vi "Actor Core_mouse down.vi"(8 "error in":errorcluster, 11 "Batch proc":refnum<class "Batch Processor.lvclass">) -> (0 "error out":errorcluster, 3 "Actor out":refnum<class "Actor.lvclass">)   [LabVIEW 2020]
doc: "LabActor main control pannel"
uses:
  <vilib>/ActorFramework/Actor/Actor.lvclass
  <vilib>/ActorFramework/Stop Msg/Stop Msg.lvclass
  LabActor Messages/Stop Measurements Command Msg/Stop Measurements Command Msg.lvclass
  Application Controller Messages/Open Waveform File Plot Msg/Open Waveform File Plot Msg.lvclass
  Plots/Plot types.ctl
  Template Module Messages/Save Configuration Msg/Save Configuration Msg.lvclass
  Template Module Messages/Restore Configuration Msg/Restore Configuration Msg.lvclass
  Batch Processor Messages/List Folder Files Msg/List Folder Files Msg.lvclass
  Batch Processor Messages/Start Batch Process Msg/Start Batch Process Msg.lvclass
  NHMFL_Core/Libraries/Queued Listbox/Queued Listbox.xctl
  Batch Processor Messages/Select Item Msg/Select Item Msg.lvclass
  Batch Processor.lvclass
  C:/GitHub/LabActor/Controllers/Application Controller/Application Controller.lvclass
  C:/GitHub/LabActor/Controllers/Process Controller/Process Controller.lvclass
  C:/GitHub/LabActor/Worker/Worker.lvclass
  C:/GitHub/LabActor/Template Module/Template Module.lvclass
  C:/Program Files/National Instruments/LabVIEW 2020/vi.lib/ActorFramework/Actor/Actor.lvclass
  C:/GitHub/LabActor/Controllers/Batch Processor/Batch Processor.lvclass
panel:
  in  "Add files  from m-file":bool
  in  "Clear files":bool
  in  "Add files":bool
  in  "Step Forward Button":bool
  out "Current file":u32
  out "Elapsed time":dbl format="%#_gs"
  in  "Configuration":T1
  in  "All files in folder":bool
  in  "About Button":bool
  in  "Clear log":bool
  out "Error log":string
  out "Monitor file":path caption="Monitor\nFile"
  in  "Exit":bool
  in  "Write cfg":bool
  in  "Read cfg":bool
  in  "View XY Plot":bool
  out "Monitor Running":bool
  in  "Stop monitor":bool
  in  "Start monitor":bool
  in  "Monitor":string[](xcontrol) caption="Processors"
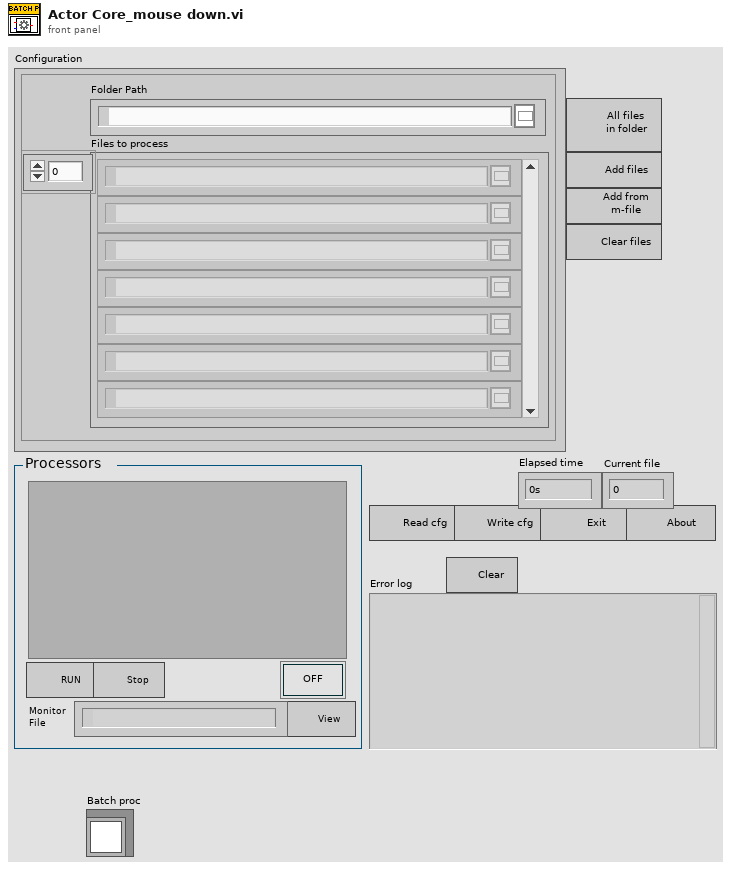
[diagram p1: front panel]
types:
  T1 = cluster{"Folder Path":path, "Files to process":path[]}
  T2 = typedef "Plot types.ctl" = enum16{"Waveform Plot", "XY Plot", "Full XY"}
  T3 = typedef "LVRectTypeDef.ctl" = cluster{"Left":i16, "Top":i16, "Right":i16, "Bottom":i16}
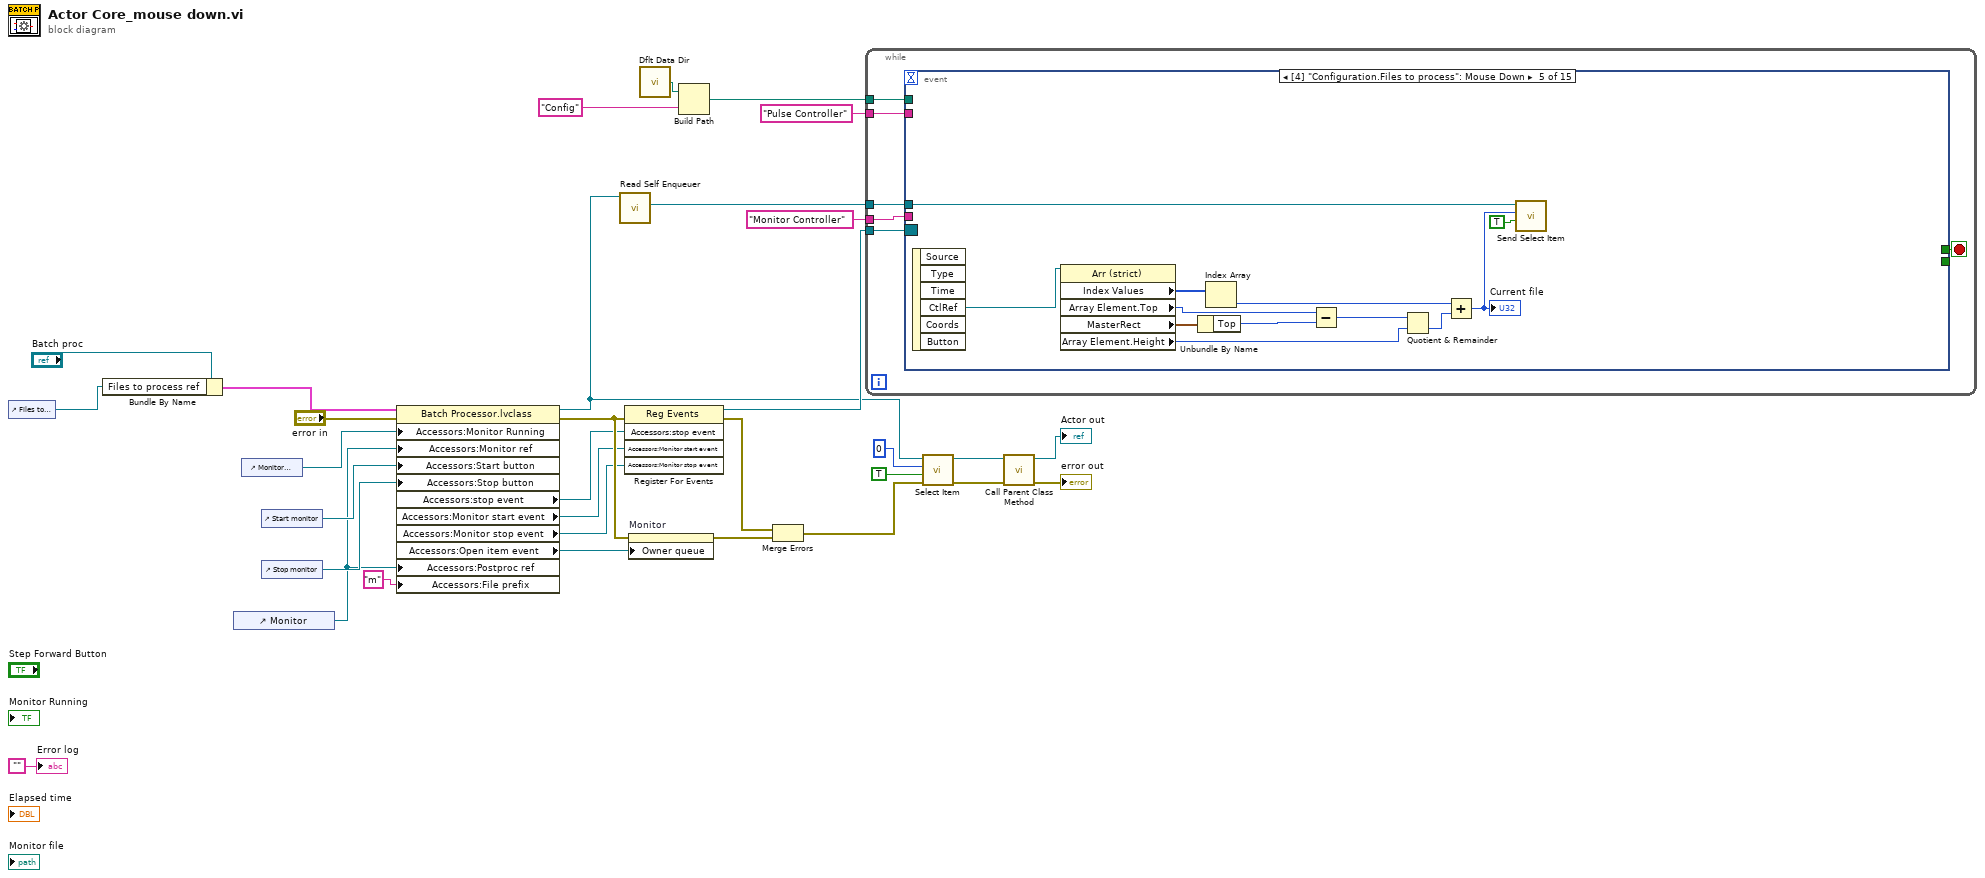
[diagram p0: block diagram]
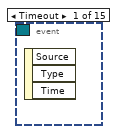
[diagram p2: hidden frame]
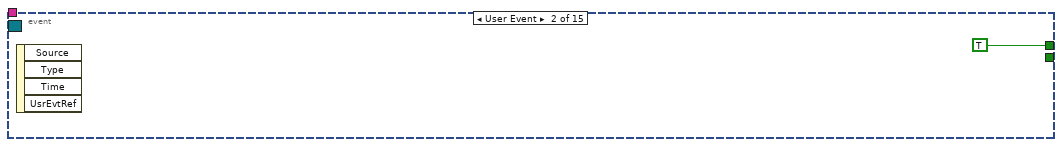
[diagram p3: hidden frame]
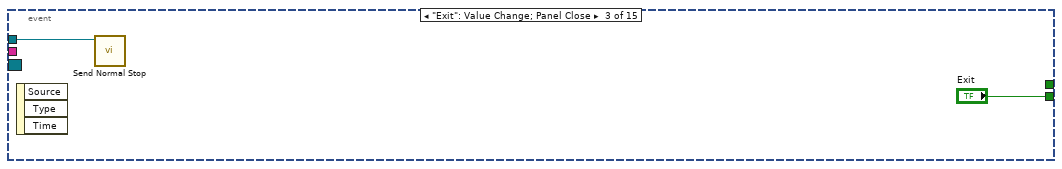
[diagram p4: hidden frame]
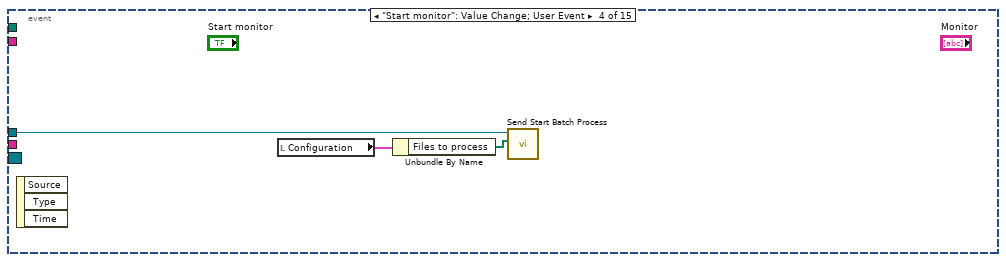
[diagram p5: hidden frame]
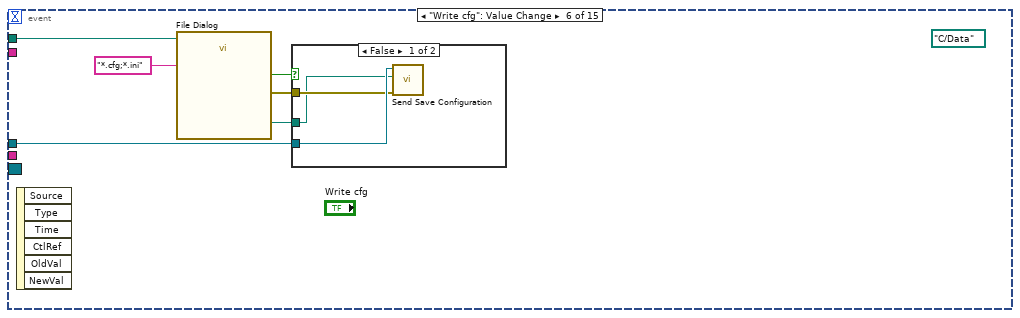
[diagram p6: hidden frame]
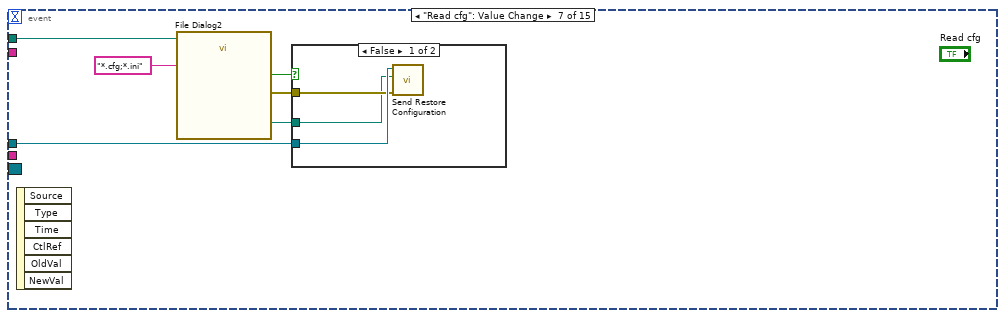
[diagram p8: hidden frame]
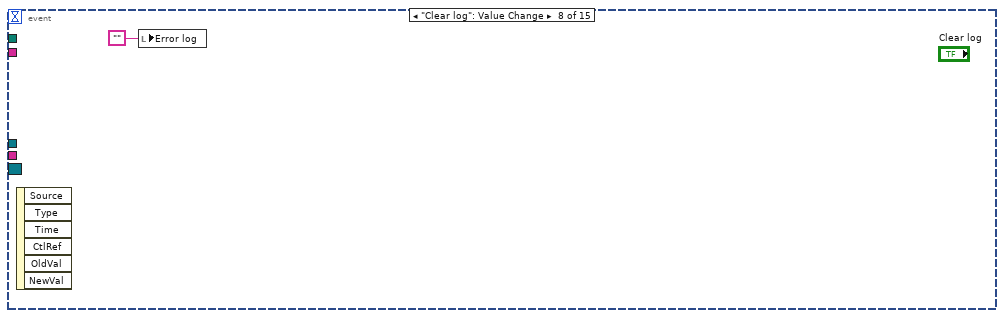
[diagram p10: hidden frame]
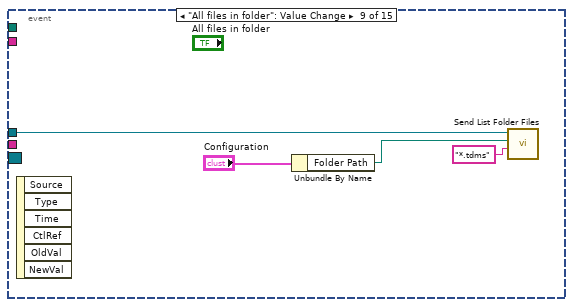
[diagram p11: hidden frame]
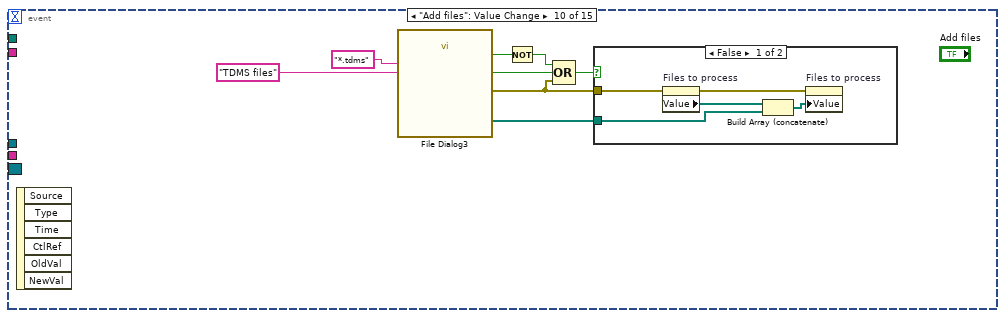
[diagram p12: hidden frame]
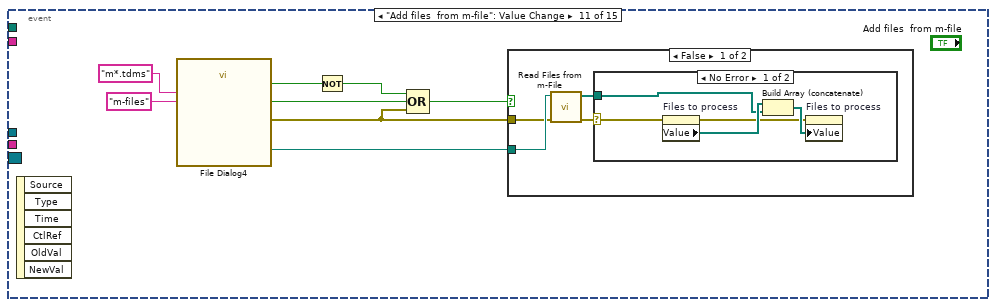
[diagram p14: hidden frame]
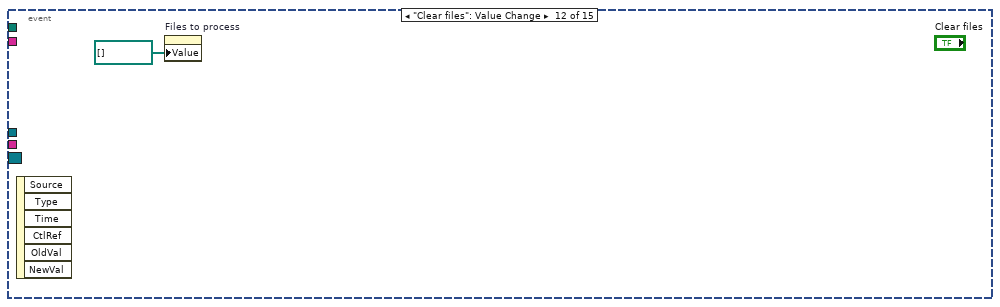
[diagram p17: hidden frame]
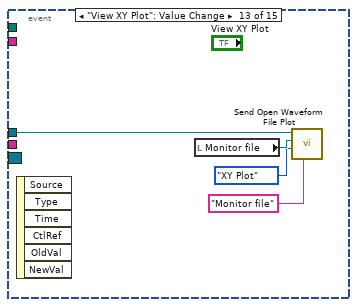
[diagram p18: hidden frame]
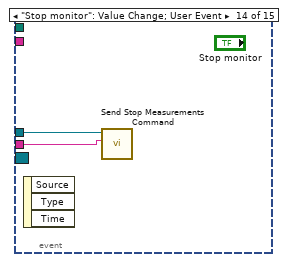
[diagram p19: hidden frame]
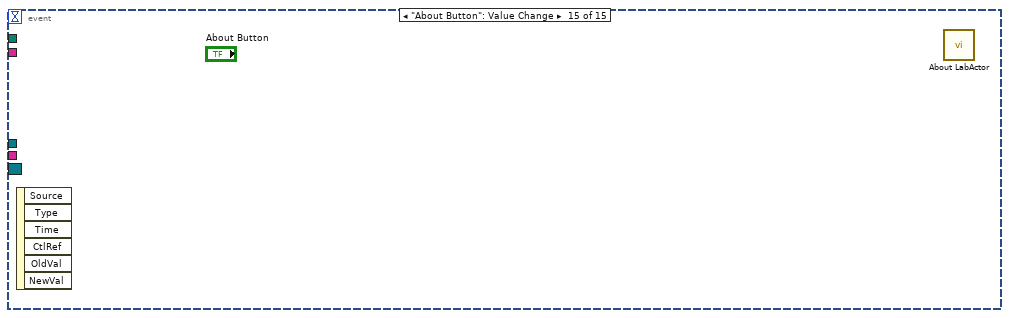
[diagram p20: hidden frame]
diagram:
  n1 = control-ref of="Files to process"() -> (w6:refnum<vi>)
  n2 = Bundle By Name(cluster="Batch proc", "Files to process ref"=w6) -> (w7:cluster{})
  n3 = control-ref of="Monitor"() -> (w12:refnum<vi>)
  n4 = control-ref of="Monitor Running"() -> (w17:refnum<vi>)
  n5 = control-ref of="Start monitor"() -> (w15:refnum<vi>)
  n6 = control-ref of="Stop monitor"() -> (w16:refnum<vi>)
  n7 = property class="Batch Processor.lvclass"(reference=w7, error in="error in", "Accessors:Monitor Running"=w17, "Accessors:Monitor ref"=w12, "Accessors:Start button"=w15, "Accessors:Stop button"=w16, "Accessors:Postproc ref"=w12, "Accessors:File prefix"="m" ("File prefix")) -> (reference out=w23:refnum<class "Batch Processor.lvclass">, error out=w26:errorcluster, "Accessors:stop event"=w18:refnum<user-event>, "Accessors:Monitor start event"=w14:refnum<user-event>, "Accessors:Monitor stop event"=w13:refnum<user-event>, "Accessors:Open item event"=w28:refnum<user-event>)
  n8 = call <vilib>:"Read Self Enqueuer.vi"("Actor"=w23) -> ("Self Enqueuer"=w22:refnum<class "Message Enqueuer.lvclass">)  [unwired: 10 in]
  n9 = register-events(error in=w26, w18, w14, w13) -> (reference out=w29:refnum<event-registration>, error out=w25:errorcluster)  [unwired: 1 in]
  n10 = property on="Monitor" class="Queued Listbox (strict)"(error in=w26, "Owner queue"=w28) -> (error out=w27:errorcluster)  [unwired: 1 in, 1 out]
  n11 = call <vilib>:"Dflt Data Dir.vi"() -> ("App:Default Data Directory"=w11:path)
  n12 = Build Path(base path=w11, name or relative path="Config") -> (appended path=w9:path)
  n13 = Merge Errors(w25, w27) -> (w4:errorcluster)
  n14 = while {
    tunnel: w29 -> [w38]
    tunnel: w22 -> [w36]
    tunnel: "Monitor Controller" ("Controller name") -> [w35]
    tunnel: "Pulse Controller" ("Item name") -> [w34]
    tunnel: w9 -> [w33]
    stop <- w37 stop-if-true
    n15 = event shown="[4] \"Configuration.Files to process\": Mouse Down" {
      selector: w38 -> [_ _ _ _ _ _ _ _ _ _ _ _ _ _ _]
      dyn-events: _ -> [_ _ _ _ _ _ _ _ _ _ _ _ _ _ _]
      timeout: _ -> [_ _ _ _ _ _ _ _ _ _ _ _ _ _ _]
      tunnel: [_ TRUE _ _ _ _ _ _ _ _ _ _ _ _ _] -> w37
      tunnel: w36 -> [_ _ w40 w44 w47 w59 w68 _ w79 _ _ _ w114 w116 _]
      tunnel: [_ _ "Exit" _ _ _ _ _ _ _ _ _ _ _ _] -> _
      tunnel: w35 -> [_ _ _ _ _ _ _ _ _ _ _ _ _ w115 _]
      tunnel: w34 -> [_ _ _ _ _ _ _ _ _ _ _ _ _ _ _]
      tunnel: w33 -> [_ _ _ _ _ w57 w66 _ _ _ _ _ _ _ _]
      event Timeout {
        n16 = event-data() -> ()  [unwired: 1 in, 3 out]
      }
      event User Event {
        n17 = event-data() -> ()  [unwired: 1 in, 4 out]
      }
      event "Exit": Value Change; Panel Close {
        n18 = event-data() -> ()  [unwired: 1 in, 3 out]
        n19 = call <vilib>:"Send Normal Stop.vi"("Message Enqueuer"=w40) -> ()  [unwired: 10 in, 1 out]
      }
      event "Start monitor": Value Change; User Event {
        n20 = event-data() -> ()  [unwired: 1 in, 3 out]
        n21 = local read "Configuration"() -> (w43:T1)
        n22 = Unbundle By Name(w43) -> ("Files to process"=w42:path[])
        n23 = call "Send Start Batch Process.vi"("Files to process"=w42, "Message Enqueuer"=w44) -> ()  [unwired: 8 in, 2 out]
      }
      event "Configuration.Files to process": Mouse Down {
        n24 = event-data() -> ("CtlRef"=w55:refnum<vi>)  [unwired: 1 in, 5 out]
        n25 = property class="Arr (strict)"(reference=w55) -> ("Index Values"=w56:u32[], "Array Element.Top"=w52:i32, "MasterRect"=w54:T3, "Array Element.Height"=w50:u32)  [unwired: 1 in, 2 out]
        n26 = Unbundle By Name(w54) -> ("Top"=w53:i16)
        n27 = Index Array(array=w56) -> (element=w49:u32)  [unwired: 1 in]
        n28 = Subtract(x=w52, y=w53) -> (x-y=w51:i32)
        n29 = Quotient & Remainder(x=w51, y=w50) -> (floor(x/y)=w48:u32)  [unwired: 1 out]
        n30 = Add(x=w49, y=w48) -> (x+y=w46:u32)
        "Current file" <- w46
        n31 = call "Send Select Item.vi"("Update internal index"=TRUE, "Item index"=w46, "Message Enqueuer"=w47) -> ()  [unwired: 7 in, 2 out]
      }
      event "Write cfg": Value Change {
        (unwired) path "C:/Data" ("start path")
        n32 = event-data() -> ()  [unwired: 1 in, 6 out]
        n33 = call "File Dialog"("start path"=w57, "pattern (all files)"="*.cfg;*.ini") -> ("selected path"=w61:path, "cancelled"=w62:bool, "error out"=w58:errorcluster)  [unwired: 10 in, 1 out]
        n34 = case shown="False" w62 {
          tunnel: w61 -> [w63 _]
          tunnel: w59 -> [w65 _]
          tunnel: w58 -> [w64 _]
          frame False {
            n35 = call "Send Save Configuration.vi"("error in (no error)"=w64, "File path"=w63, "Message Enqueuer"=w65) -> ()  [unwired: 7 in, 2 out]
          }
          frame True {
          }
        }
      }
      event "Read cfg": Value Change {
        n36 = event-data() -> ()  [unwired: 1 in, 6 out]
        n37 = call "File Dialog2"("start path"=w66, "pattern (all files)"="*.cfg;*.ini") -> ("selected path"=w71:path, "cancelled"=w67:bool, "error out"=w69:errorcluster)  [unwired: 10 in, 1 out]
        n38 = case shown="False" w67 {
          tunnel: w71 -> [w72 _]
          tunnel: w68 -> [w74 _]
          tunnel: w69 -> [w73 _]
          frame False {
            n39 = call "Send Restore Configuration.vi"("error in (no error)"=w73, "File path"=w72, "Message Enqueuer"=w74) -> ()  [unwired: 7 in, 2 out]
          }
          frame True {
          }
        }
      }
      event "Clear log": Value Change {
        n40 = event-data() -> ()  [unwired: 1 in, 6 out]
        n41 = local write "Error log"("" ("Error log")) -> ()
      }
      event "All files in folder": Value Change {
        n42 = event-data() -> ()  [unwired: 1 in, 6 out]
        n43 = Unbundle By Name("Configuration") -> ("Folder Path"=w77:path)
        n44 = call "Send List Folder Files.vi"("Pattern"="*.tdms", "Folder Path"=w77, "Message Enqueuer"=w79) -> ()  [unwired: 7 in, 2 out]
      }
      event "Add files": Value Change {
        n45 = event-data() -> ()  [unwired: 1 in, 6 out]
        n46 = call "File Dialog3"("pattern (all files)"="*.tdms", "pattern label"="TDMS files") -> ("selected paths"=w82:path[], "exists"=w81:bool, "cancelled"=w84:bool, "error out"=w83:errorcluster)  [unwired: 10 in]
        n47 = Not(x=w81) -> (.not. x?=w80:bool)
        n48 = Compound Arithmetic op=OR(w80, w84, w83) -> (w85:bool)
        n49 = case shown="False" w85 {
          tunnel: w83 -> [w91 _]
          tunnel: w82 -> [w89 _]
          frame False {
            n50 = property on="Files to process" class="Arr (strict)"(error in=w91) -> (error out=w88:errorcluster, "Value"=w92:path[])  [unwired: 1 in, 1 out]
            n51 = Build Array (concatenate)(w92, w89) -> (w90:path[])
            n52 = property on="Files to process" class="Arr (strict)"(error in=w88, "Value"=w90) -> ()  [unwired: 1 in, 2 out]
          }
          frame True {
          }
        }
      }
      event "Add files  from m-file": Value Change {
        n53 = event-data() -> ()  [unwired: 1 in, 6 out]
        n54 = call "File Dialog4"("pattern (all files)"="m*.tdms", "pattern label"="m-files") -> ("selected path"=w93:path, "exists"=w95:bool, "cancelled"=w97:bool, "error out"=w96:errorcluster)  [unwired: 10 in]
        n55 = Not(x=w95) -> (.not. x?=w94:bool)
        n56 = Compound Arithmetic op=OR(w94, w97, w96) -> (w98:bool)
        n57 = case shown="False" w98 {
          tunnel: w96 -> [w101 _]
          tunnel: w93 -> [w104 _]
          frame False {
            n58 = call "Read Files from m-File.vi"("error in"=w101, "File Path"=w104) -> ("error out"=w102:errorcluster, "Paths"=w103:path[])  [unwired: 8 in]
            n59 = case shown="No Error" w102 {
              selector: w102 -> [w105 _]
              tunnel: w103 -> [w106 _]
              frame No Error {
                n60 = property on="Files to process" class="Arr (strict)"(error in=w105) -> (error out=w107:errorcluster, "Value"=w109:path[])  [unwired: 1 in, 1 out]
                n61 = Build Array (concatenate)(w109, w106) -> (w108:path[])
                n62 = property on="Files to process" class="Arr (strict)"(error in=w107, "Value"=w108) -> ()  [unwired: 1 in, 2 out]
              }
              frame Error {
              }
            }
          }
          frame True {
          }
        }
      }
      event "Clear files": Value Change {
        n63 = event-data() -> ()  [unwired: 1 in, 6 out]
        n64 = property on="Files to process" class="Arr (strict)"("Value"=path[] []) -> ()  [unwired: 2 in, 2 out]
      }
      event "View XY Plot": Value Change {
        n65 = event-data() -> ()  [unwired: 1 in, 6 out]
        n66 = local read "Monitor file"() -> (w113:path)
        n67 = call "Send Open Waveform File Plot.vi"("Plot group"="Monitor file" ("Control Name"), "Plot type"=Plot_types."XY Plot", "File Path Control"=w113, "Message Enqueuer"=w114) -> ()  [unwired: 6 in, 2 out]
      }
      event "Stop monitor": Value Change; User Event {
        n68 = event-data() -> ()  [unwired: 1 in, 3 out]
        n69 = call "Send Stop Measurements Command.vi"("Measurement Controller"=w115, "Message Enqueuer"=w116) -> ()  [unwired: 8 in, 2 out]
      }
      event "About Button": Value Change {
        n70 = event-data() -> ()  [unwired: 1 in, 6 out]
        n71 = call "About LabActor.vi"() -> ()  [unwired: 11 in, 1 out]
      }
    }
  }
  n72 = call-dynamic "Select Item.vi"("error in (no error)"=w4, "Update internal index"=TRUE, "Item index"=0, "Batch Processor in"=w23) -> ("error out"=w3:errorcluster, "Batch Processor out"=w5:refnum<class "Batch Processor.lvclass">)  [unwired: 6 in]
  n73 = call-parent "Call Parent Class Method"("error in"=w3, "Measure Object in"=w5) -> ("error out"=→"error out":errorcluster, "Actor out"=→"Actor out":refnum<class "Actor.lvclass">)  [unwired: 8 in]
  "Error log" <- "" ("Error log")
